vi "UTILITY Array Get 1D Row From 2D String.vi"(0 "all rows":string[][](array[string]), 7 "row index":i32) -> (4 "row":string[](array[string]))   [LabVIEW 2016]
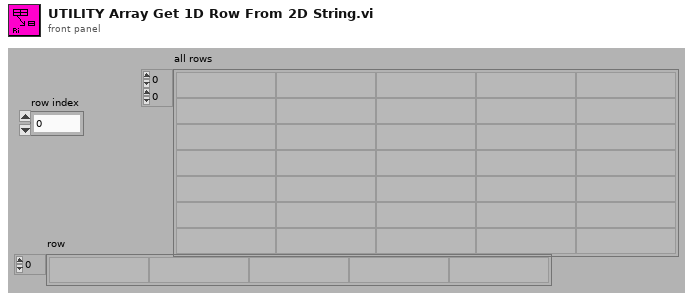
[diagram p1: front panel]
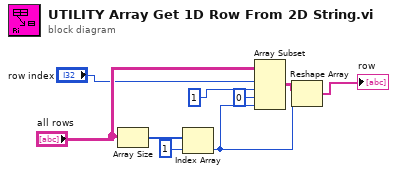
[diagram p0: block diagram]
diagram:
  n1 = Array Size(array="all rows") -> (size(s)=w8:i32[])
  n2 = Index Array(array=w8, index=1) -> (element=w3:i32)
  n3 = Array Subset(array="all rows", index (row)="row index", length (row)=1 ("length"), index (col)=0 ("index"), length (col)=w3) -> (w9:string[][])
  n4 = Reshape Array(w9, w3) -> (→"row":string[])
